vi "Scale_0_1 (SubVI).vi"(11 "BLine D":dbl[](array[numeric])) -> (3 "Array":dbl[](array[numeric]))   [LabVIEW 2017]
uses:
  <vilib>/Analysis/NI_AALBase.lvlib
  <vilib>/Analysis/baseanly.llb/Scale 1D.vi
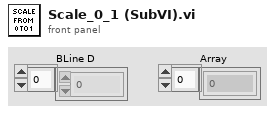
[diagram p1: front panel]
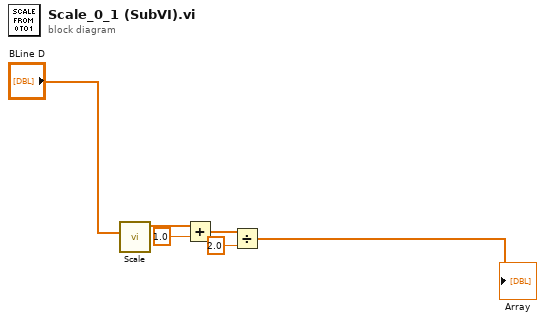
[diagram p0: block diagram]
diagram:
  n1 = call-poly <vilib>:"Scale.vi"("X"="BLine D") -> ("Y=(X-offset)/scale"=w1:dbl[])  [unwired: 3 out]
  n2 = Add(x=w1, y=1.0) -> (x+y=w3:dbl[])
  n3 = Divide(x=w3, y=2.0) -> (x/y=→"Array":dbl[])
